vi "onCreateListener.vi"(6 "timeout (ms)":i32=100, 8 "error in (no error)":errorcluster, 10 "Configuration":refnum<class "LocalQueueConnection.lvclass">) -> (0 "error out":errorcluster, 3 "Listener":refnum<class "Connection.lvclass">)   [LabVIEW 2013, in "MQTT_Queue.lvlib" / "LocalQueueConnection.lvclass"]
uses:
  LocalQueueConnection.lvclass
  <vilib>/LabVIEW Open Source Project/MQTT Connection/MQTT_Connection/Connection/Connection.lvclass
  LocalQueueConnection.lvclass/LocalQueueConnection.ctl
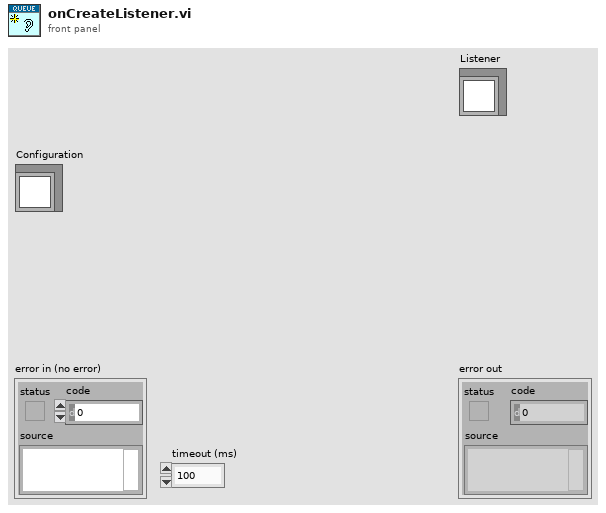
[diagram p1: front panel]
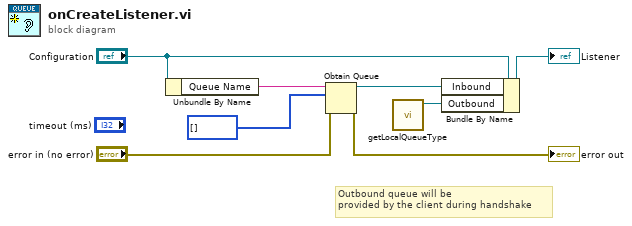
[diagram p0: block diagram]
diagram:
  # "Outbound queue will be\nprovided by the client during handshake"
  n1 = Unbundle By Name("Configuration") -> ("Queue Name"=w2:string)
  n2 = Obtain Queue(name (unnamed)=w2, element data type=u8[] [] ("Bytes Stream"), error in (no error)="error in (no error)") -> (queue out=w7:refnum<queue>, error out=→"error out":errorcluster)  [unwired: 2 in, 1 out]
  n3 = call "getLocalQueueType.vi"() -> ("Queue Type"=w1:refnum<queue>)  [unwired: 11 in]
  n4 = Bundle By Name(cluster="Configuration", "Inbound"=w7, "Outbound"=w1) -> (→"Listener":refnum<class "LocalQueueConnection.lvclass">)
